vi "Pre Launch Init.vi"(11 "Contador_Actor_Interface in":refnum<class "Contador_Actor_Interface.lvclass">) -> (0 "error out":errorcluster, 3 "Contador_Actor_Interface out":refnum<class "Contador_Actor_Interface.lvclass">)   [LabVIEW 2019, in "Contador_Actor_Interface.lvlib" / "Contador_Actor_Interface.lvclass"]
doc: "(<B>Filename</B>: Actor Framework.lvlib:Actor.lvclass:Pre Launch Init.vi)\n\nDefines behavior that occurs after the Launch Nested Actor method is invoked but before the actor's Actor Core method begins running.\n\nBy default, this method does nothing. A descendant class may override it to define behavior."
uses:
  Contador_Actor_Interface.lvclass
  <vilib>/ActorFramework/Actor/Actor.lvclass
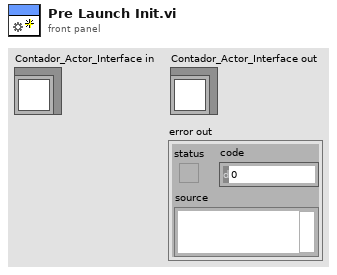
[diagram p1: front panel]
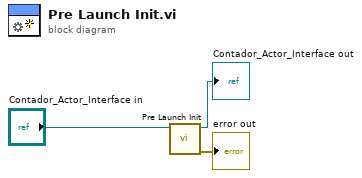
[diagram p0: block diagram]
diagram:
  n1 = call-parent "Pre Launch Init.vi"("Actor in"="Contador_Actor_Interface in") -> ("error out"=→"error out":errorcluster, "Actor out"=→"Contador_Actor_Interface out":refnum<class "Contador_Actor_Interface.lvclass">)  [unwired: 9 in]
